vi "hind brain 2.vi"() -> ()   [LabVIEW 2011, in "Hindbrain Demo.lvrbt"]
uses:
  Hindbrain Demo.lvrbt
  <vilib>/NXT/Block Support/HWPage.SensorType.ctl
  <vilib>/NXT/Block Support/HWPage.SensorMode.ctl
  <vilib>/NXT/Block Support/NXT_InputPort.ctl
  <vilib>/addons/mindsensors.com_LVEE_Toolkit_V1.23/mindsensors.com LVEE Toolkit/Dual/NXTServo-DM.vi
  <vilib>/NXT/Dual Mode Library/Sensors/Color_None.vi
panel:
  in  "Input of NXTServo 2":T1={"Servo Number"=2, "Position"=1500, "Speed"=0} {"Speed" step=1 scale=0.0..255.0; "Position" min=500 max=2500 step=1 scale=500.0..2500.0; "Servo Number" min=1 max=8 step=1}
  out "Output of NXTServo 2":cluster{"Voltage":u8, "Status":bool}
  in  "stop":bool
  in  "Input of NXTServo":T1={"Servo Number"=1, "Position"=1500, "Speed"=0} {"Speed" step=1 scale=0.0..255.0; "Position" min=500 max=2500 step=1 scale=500.0..2500.0; "Servo Number" min=1 max=8 step=1}
  out "Output of NXTServo":cluster{"Voltage":u8, "Status":bool}
  out "Pressed?":bool caption="Switch\nPressed?"
  out "Light Intensity":i16 caption="Scaled Value"
  out "Blink":bool
  out "Battery mv":i32
  out "Scaled Value":i16
  out "Left?":bool
  out "Right?":bool
  out "Front?":bool
  out "Stuff?":bool
  # "This is a demonstration of how to sense and acturate devices on the LEGO NXT brick.\nThe connections to the NXT brick are as follows:\nNOTHING IS CONNECTED TO PORTS A, B AND C.\nPort 1 has the Mindsensor NXTServo\nPort 2 has the LEGO Color Sensor\nPort 3 has the LEGO Switch\nPort 4 and the Mindsensor NXTSumoEyes-v3."
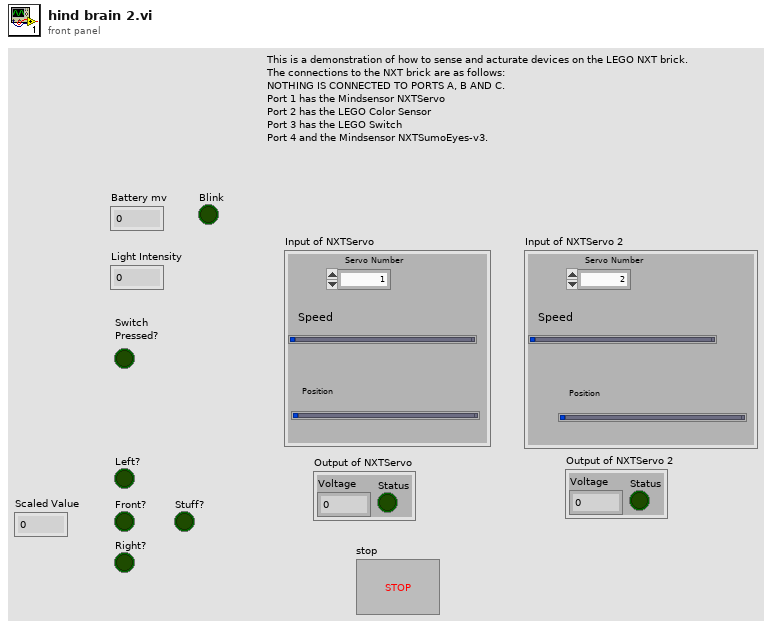
[diagram p1: front panel]
types:
  T1 = cluster{"Servo Number":u8, "Position":u16, "Speed":u8}
  T2 = typedef "NXT_InputPort.ctl" = u8
  T3 = typedef "HWPage.SensorType.ctl" = u8
  T4 = typedef "HWPage.SensorMode.ctl" = u8
  T5 = typedef "LVHSConnector.ctl" = cluster{"Hardware":string, "Flattened String":string}
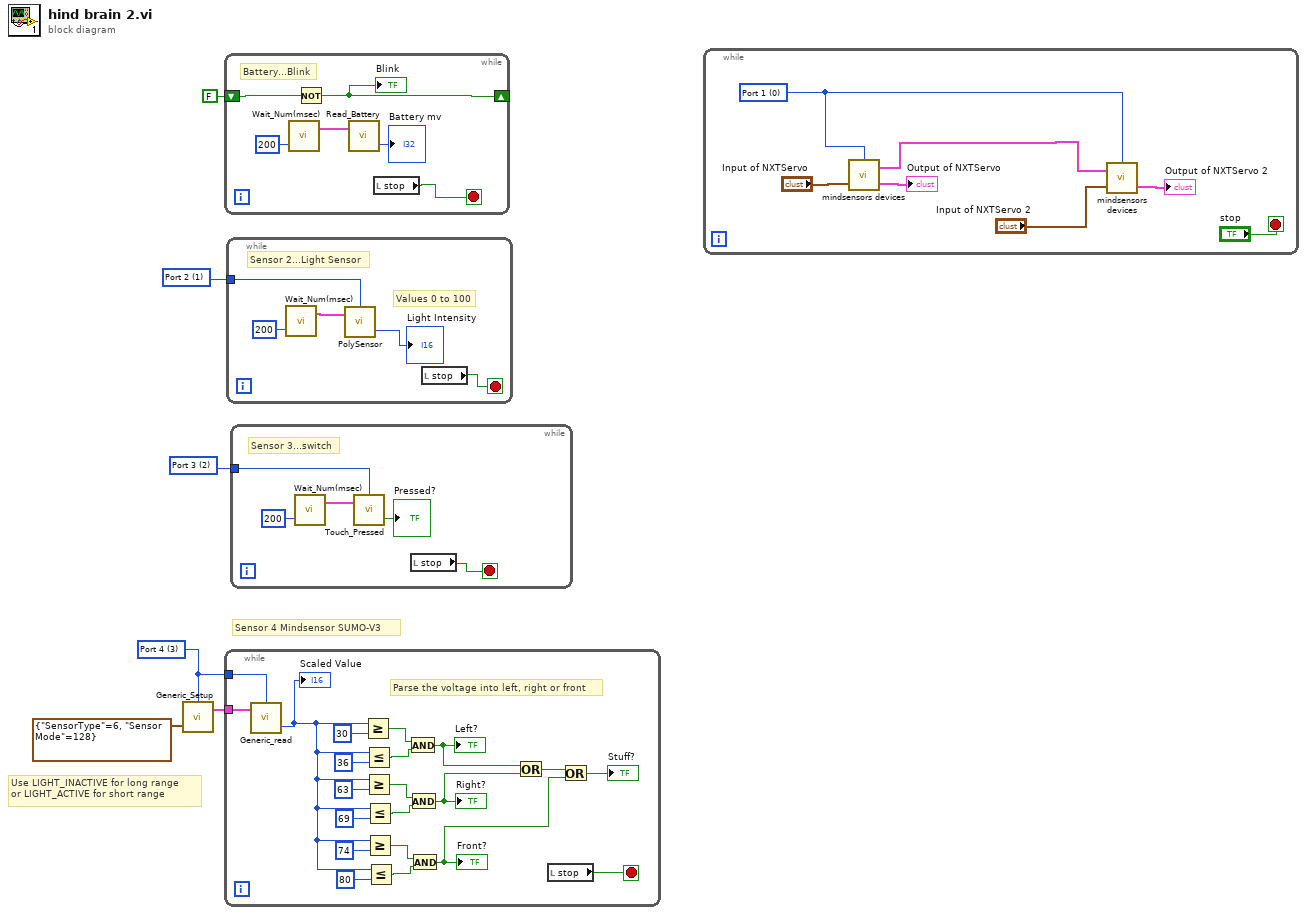
[diagram p0: block diagram]
diagram:
  w1 = T2 2 items=["Port 1", "Port 2", "Port 3", "Port 4"] ("Port (Port 1)")
  w2 = T2 1 items=["Port 1", "Port 2", "Port 3", "Port 4"] ("Port (Port 3)")
  w3 = T2 3 items=["Port 1", "Port 2", "Port 3", "Port 4"] ("Port")
  # "Sensor 4 Mindsensor SUMO-V3"
  # "Use LIGHT_INACTIVE for long range\nor LIGHT_ACTIVE for short range"
  n1 = call <vilib>:"Generic_Setup.vi"("Sensor Setup"=cluster{"SensorType":T3, "Sensor Mode":T4} {"SensorType"=6, "Sensor Mode"=128}, "Port"=w3) -> ("NXT"=w6:T5)  [unwired: 1 in, 1 out]
  n2 = while {
    shift-right: [w8] -> _
    shift-left: FALSE -> [w9]
    stop <- w10 stop-if-true
    # "Battery...Blink"
    n3 = call <vilib>:"Wait_Num(msec).vi"("Time (100 msec)"=u32 200) -> ("NXT"=w11:T5)  [unwired: 3 in]
    n4 = Not(x=w9) -> (.not. x?=w8:bool)
    "Blink" <- w8
    n5 = call <vilib>:"Read_Battery.vi"("NXT"=w11) -> ("millivolts"=→"Battery mv":i32)  [unwired: 2 in, 1 out]
    n6 = local read "stop"() -> (w10:bool)
  }
  n7 = while {
    tunnel: w3 -> [w33]
    tunnel: w6 -> [w32]
    stop <- w13 stop-if-true
    # "Parse the voltage into left, right or front"
    n8 = call <vilib>:"Generic_read.vi"("NXT"=w32, "Port (Port 3)"=w33) -> ("Scaled Value"=w19:i16)  [unwired: 2 out]
    "Scaled Value" <- w19
    n9 = Greater Or Equal?(x=w19, y=i16 30) -> (x >= y?=w29:bool)
    n10 = Less Or Equal?(x=w19, y=i16 36) -> (x <= y?=w28:bool)
    n11 = Greater Or Equal?(x=w19, y=i16 63) -> (x >= y?=w26:bool)
    n12 = Less Or Equal?(x=w19, y=i16 69) -> (x <= y?=w27:bool)
    n13 = Greater Or Equal?(x=w19, y=i16 74) -> (x >= y?=w22:bool)
    n14 = Less Or Equal?(x=w19, y=i16 80) -> (x <= y?=w23:bool)
    n15 = And(x=w29, y=w28) -> (x .and. y?=w18:bool)
    "Left?" <- w18
    n16 = And(x=w26, y=w27) -> (x .and. y?=w17:bool)
    "Right?" <- w17
    n17 = And(x=w22, y=w23) -> (x .and. y?=w15:bool)
    "Front?" <- w15
    n18 = Or(x=w18, y=w17) -> (x .or. y?=w16:bool)
    n19 = local read "stop"() -> (w13:bool)
    n20 = Or(x=w16, y=w15) -> (x .or. y?=→"Stuff?":bool)
  }
  n21 = while {
    tunnel: w2 -> [w34]
    stop <- w37 stop-if-true
    # "Values 0 to 100"
    # "Sensor 2...Light Sensor"
    n22 = call <vilib>:"Wait_Num(msec).vi"("Time (100 msec)"=u32 200) -> ("NXT"=w36:T5)  [unwired: 3 in]
    n23 = call-poly <vilib>:"PolySensor.vi"("NXT"=w36, "Port (Port 3)"=w34) -> ("Intensity"=→"Light Intensity":i16)  [unwired: 1 in, 1 out]
    n24 = local read "stop"() -> (w37:bool)
  }
  n25 = while {
    tunnel: w1 -> [w40]
    stop <- w41 stop-if-true
    # "Sensor 3...switch"
    n26 = call <vilib>:"Wait_Num(msec).vi"("Time (100 msec)"=u32 200) -> ("NXT"=w42:T5)  [unwired: 3 in]
    n27 = call <vilib>:"Touch_Pressed.vi"("NXT"=w42, "Port (Port 1)"=w40) -> ("Yes / No"=→"Pressed?":bool)  [unwired: 1 in, 1 out]
    n28 = local read "stop"() -> (w41:bool)
  }
  n29 = while {
    stop <- "stop" stop-if-true
    w44 = T2 0 items=["Port 1", "Port 2", "Port 3", "Port 4"] ("Input Port")
    n30 = call-poly <vilib>:"mindsensors devices.vi"("Input of NXTServo"="Input of NXTServo", "Input Port"=w44) -> ("Output of NXTServo"=→"Output of NXTServo":cluster{"Voltage":u8, "Status":bool}, "NXT dup"=w45:T5)  [unwired: 1 in]
    n31 = call-poly <vilib>:"mindsensors devices.vi"("Input of NXTServo"="Input of NXTServo 2", "NXT"=w45, "Input Port"=w44) -> ("Output of NXTServo"=→"Output of NXTServo 2":cluster{"Voltage":u8, "Status":bool})  [unwired: 1 out]
  }
